vi "PrimaryInterfaceGetVariableValue.vi"(8 "Variable":refnum<k24>, 11 "error in":errorcluster) -> (0 "Value":T1, 3 "error out":errorcluster)   [LabVIEW 2022 SP3, in "UnderAutomation.UniversalRobots.lvlib"]
uses:
  UnderAutomation.UniversalRobots.lvlib
  C:/Users/fg/Documents/UniversalRobots.vi/LabVIEW_2023/UnderAutomation.UniversalRobots/lib/UnderAutomation.UniversalRobots.dll
  LabVIEW_2023/UnderAutomation.UniversalRobots/lib/UnderAutomation.UniversalRobots.dll
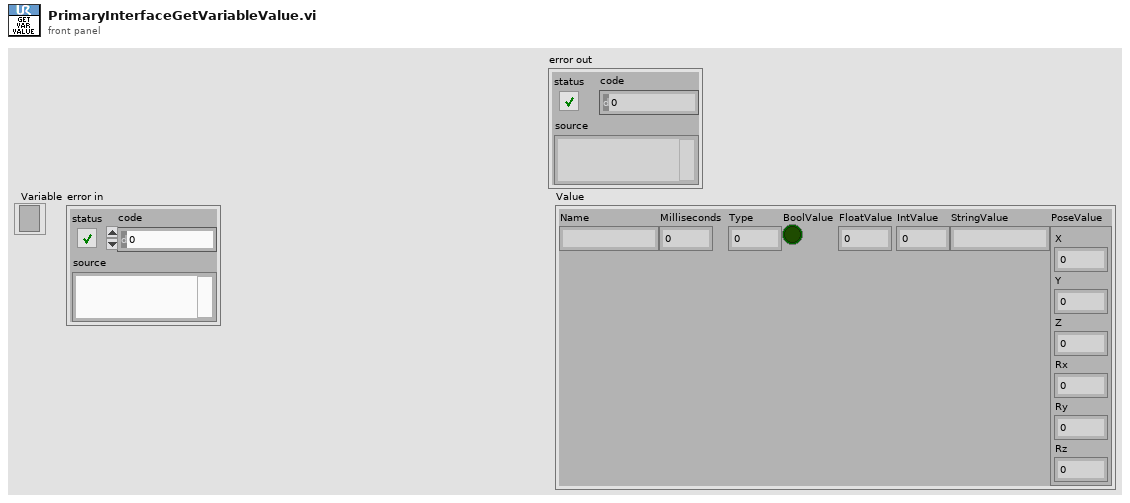
[diagram p1: front panel]
types:
  T1 = cluster{"Name":string, "Milliseconds":i32, "Type":i32, "BoolValue":bool, "FloatValue":sgl, "IntValue":i32, "StringValue":string, "PoseValue":cluster{"X":dbl, "Y":dbl, "Z":dbl, "Rx":dbl, "Ry":dbl, "Rz":dbl}}
  T2 = cluster{"X":dbl, "Y":dbl, "Z":dbl, "Rx":dbl, "Ry":dbl, "Rz":dbl}
  T3 = cluster{"Name":string, "Milliseconds":i32, "Type":i32, "ToBool":bool, "ToFloat":sgl, "ToInt":i32, "ToString":string, cluster{"X":dbl, "Y":dbl, "Z":dbl, "Rx":dbl, "Ry":dbl, "Rz":dbl}}
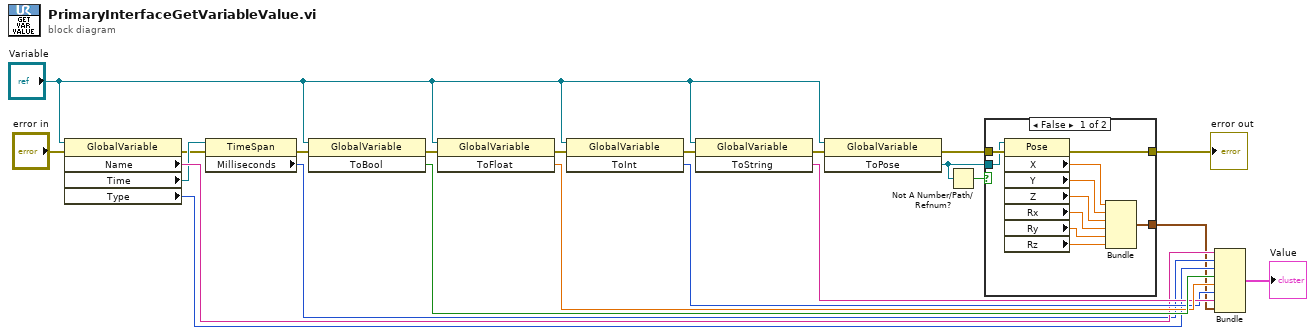
[diagram p0: block diagram]
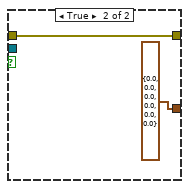
[diagram p2: hidden frame]
diagram:
  n1 = property class="GlobalVariable"(reference="Variable", error in="error in") -> (error out=w11:errorcluster, "Name"=w18:string, "Time"=w16:refnum<k24>, "Type"=w17:i32)  [unwired: 1 out]
  n2 = property class="TimeSpan"(reference=w16, error in=w11) -> (error out=w10:errorcluster, "Milliseconds"=w15:i32)  [unwired: 1 out]
  n3 = invoke class="GlobalVariable" method="ToBool"(reference="Variable", error in=w10) -> (error out=w9:errorcluster, "ToBool"=w22:bool)  [unwired: 1 in, 1 out]
  n4 = invoke class="GlobalVariable" method="ToFloat"(reference="Variable", error in=w9) -> (error out=w8:errorcluster, "ToFloat"=w21:sgl)  [unwired: 1 in, 1 out]
  n5 = invoke class="GlobalVariable" method="ToInt"(reference="Variable", error in=w8) -> (error out=w7:errorcluster, "ToInt"=w19:i32)  [unwired: 1 in, 1 out]
  n6 = invoke class="GlobalVariable" method="ToString"(reference="Variable", error in=w7) -> (error out=w6:errorcluster, "ToString"=w20:string)  [unwired: 1 in, 1 out]
  n7 = invoke class="GlobalVariable" method="ToPose"(reference="Variable", error in=w6) -> (error out=w5:errorcluster, "ToPose"=w1:refnum<k24>)  [unwired: 1 in, 1 out]
  n8 = Not A Number/Path/Refnum?(number/path/refnum=w1) -> (NaN/Path/Refnum?=w2:bool)
  n9 = case shown="False" w2 {
    tunnel: w5 -> [w26 w34]
    tunnel: [w25 T2 {"X"=0.0, "Y"=0.0, "Z"=0.0, "Rx"=0.0, "Ry"=0.0, "Rz"=0.0}] -> w4
    tunnel: [w24 w34] -> w3
    tunnel: w1 -> [w23 _]
    frame False {
      n10 = property class="Pose"(reference=w23, error in=w26) -> (error out=w24:errorcluster, "X"=w27:dbl, "Y"=w28:dbl, "Z"=w29:dbl, "Rx"=w30:dbl, "Ry"=w31:dbl, "Rz"=w32:dbl)  [unwired: 1 out]
      n11 = Bundle("X"=w27, "Y"=w28, "Z"=w29, "Rx"=w30, "Ry"=w31, "Rz"=w32) -> (w25:T2)  [unwired: 1 in]
    }
    frame True {
    }
  }
  "error out" <- w3
  n12 = Bundle("Name"=w18, "Milliseconds"=w15, "Type"=w17, "ToBool"=w22, "ToFloat"=w21, "ToInt"=w19, "ToString"=w20, w4) -> (→"Value":T3)  [unwired: 1 in]
